vi "Teleop.vi"(8 "Enum In":enum16{"Scale", "Switch", "Intake", "Reserve"}(ring), 10 "Match Info":T1={"Autonomous Elapsed Seconds"=0.0, "TeleOp Elapsed Seconds"=0.0, "Disabled Elapsed Seconds"=0.0, "Visited Autonomous"=FALSE, "Visited TeleOp"=FALSE, "Visited Disabled"=FALSE, "Autonomous Settings"={"Autonomous Style"=enum."Independent", "VI Refnum"=refnum}}, 11 "Call Context":T2) -> (0 "Enum Out":enum16{"Scale", "Switch", "Intake", "Reserve"}(ring))   [LabVIEW 2017]
doc: "This VI is called for each enabled TeleOp packet received from the DS. It is typically used to read from joysticks and other inputs and update I/O or setpoints for timed control loops. It should complete and return within 20 milliseconds or risk missing DS packets."
uses:
  <vilib>/Rock Robotics/WPI/DriverStation/WPI_DriverStationDerivedRobotMode.ctl
  <vilib>/Rock Robotics/WPI/DriverStation/WPI_DriverStationMatch Info.ctl
  9a3754dc-426d-418a-b166-45fb967c4ccf.vi
  c9379947-65ce-468e-b721-daf5d8b91ee4.vi
  b6a63361-7184-4aa3-88ad-815ff18ec719.vi
  9926fa97-c3d7-4492-8b20-f5ff4f16c79e.vi
  7ab30a6b-1479-45e7-bda8-42199c1e9ef9.vi
  <vilib>/Rock Robotics/WPI/Utilities/WPI_GetSetVariantRefNum.vi
  <vilib>/Rock Robotics/WPI/Joystick/WPI_JoystickArcadeMapping.vi
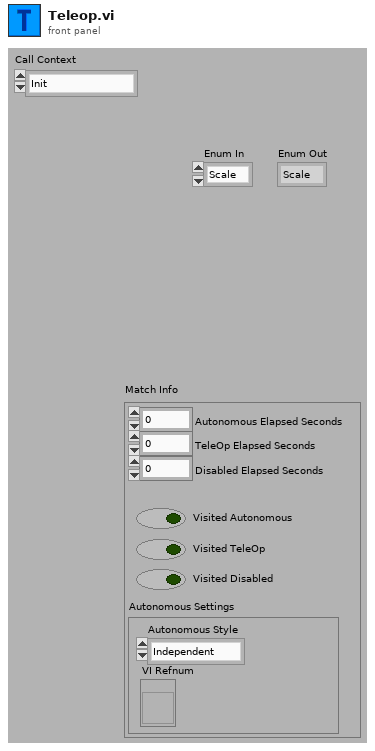
[diagram p1: front panel]
types:
  T1 = typedef "WPI_DriverStationMatch Info.ctl" = cluster{"Autonomous Elapsed Seconds":dbl, "TeleOp Elapsed Seconds":dbl, "Disabled Elapsed Seconds":dbl, "Visited Autonomous":bool, "Visited TeleOp":bool, "Visited Disabled":bool, "Autonomous Settings":cluster{"Autonomous Style":enum16{"Iterative", "Independent"}, "VI Refnum":refnum<vi>}}
  T2 = typedef "WPI_DriverStationDerivedRobotMode.ctl" = enum16{"Init", "Execute", "Stop"}
  T3 = typedef "WPI_JoystickDevRef.ctl" = cluster{"Device":T4}
  T4 = typedef "WPI_JoystickDeviceEnum.ctl" = enum16{"USB 0", "USB 1", "USB 2", "USB 3", "USB 4", "USB 5"}
  T5 = cluster{"Buttons[0]":bool, "Buttons[1]":bool, "Buttons[2]":bool, "Buttons[3]":bool, "Buttons[4]":bool, "Buttons[5]":bool, "Buttons[6]":bool, "Buttons[7]":bool, "Buttons[8]":bool}
  T6 = cluster{"POVs[0]":i16, "POVs[1]":i16, "POVs[2]":i16, "POVs[3]":i16, "POVs[4]":i16, "POVs[5]":i16, "POVs[6]":i16, "POVs[7]":i16, "POVs[8]":i16}
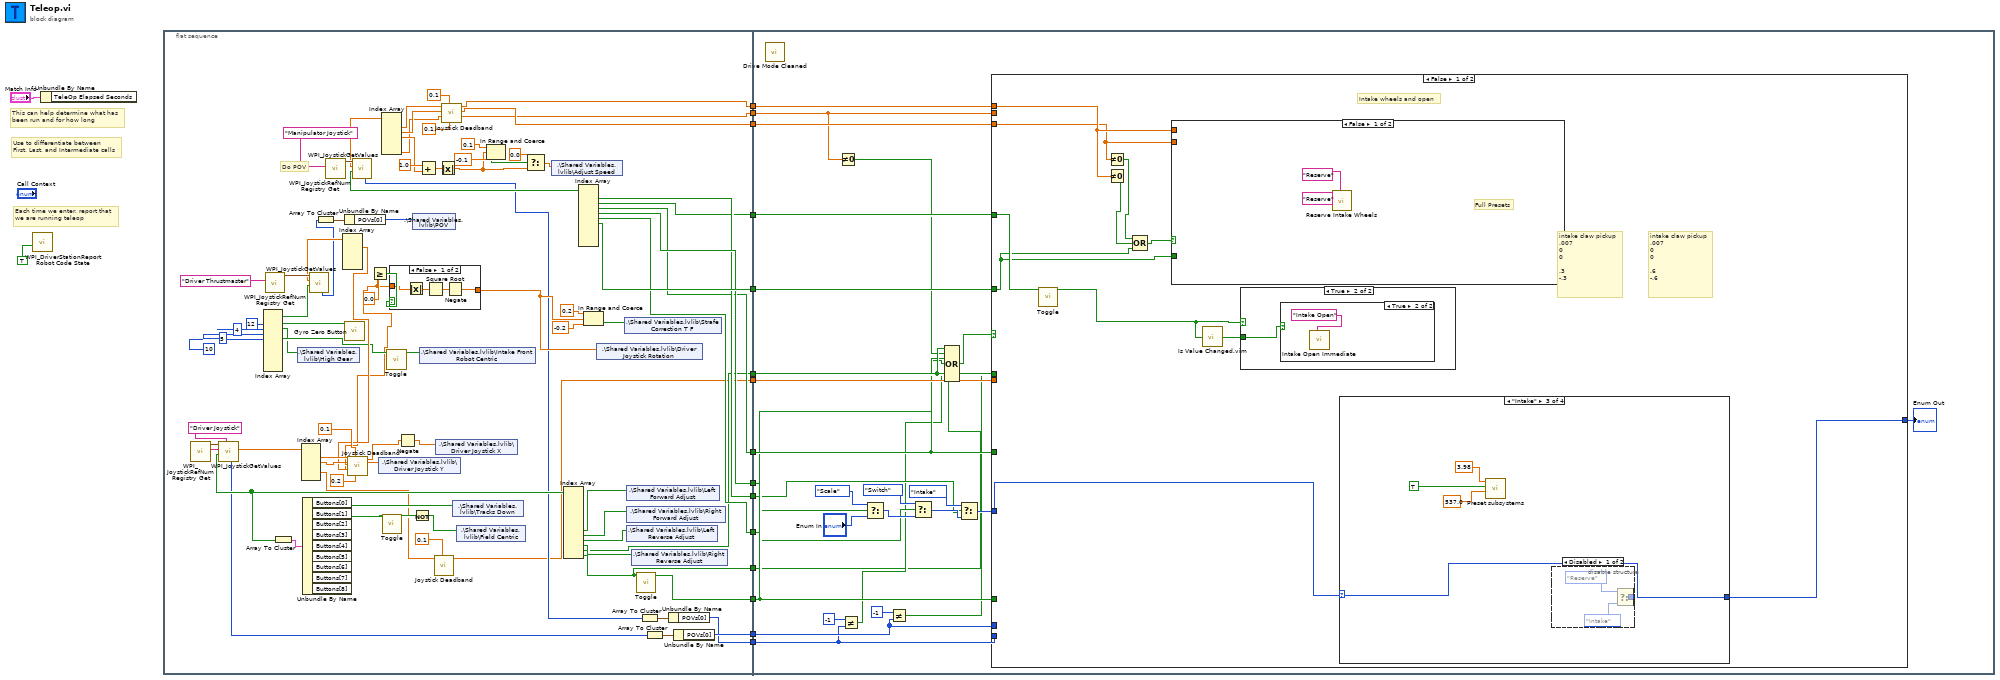
[diagram p0: block diagram]
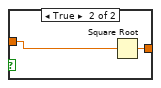
[diagram p2: hidden frame]
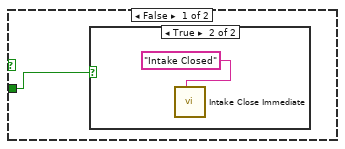
[diagram p3: hidden frame]
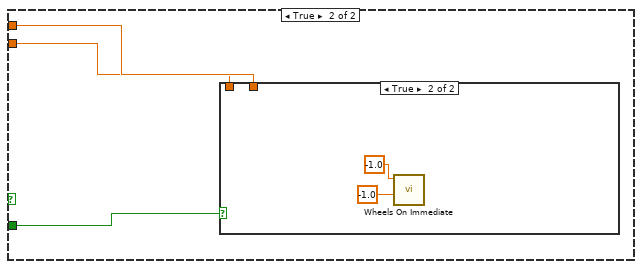
[diagram p6: hidden frame]
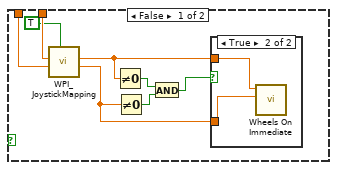
[diagram p7: hidden frame]
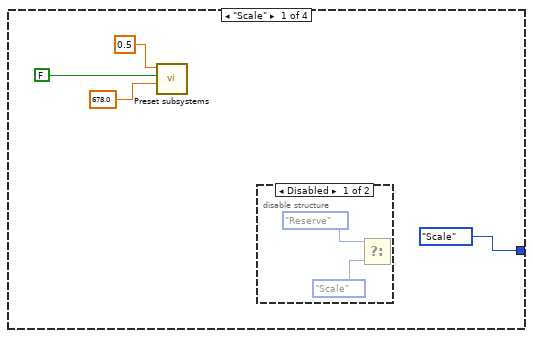
[diagram p9: hidden frame]
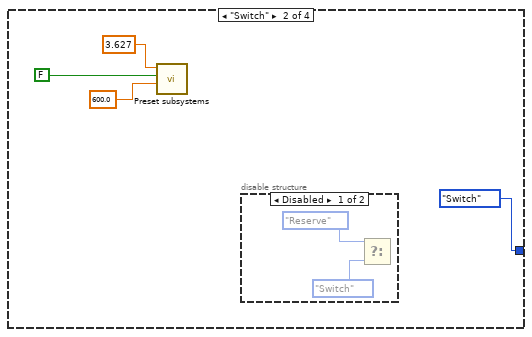
[diagram p11: hidden frame]
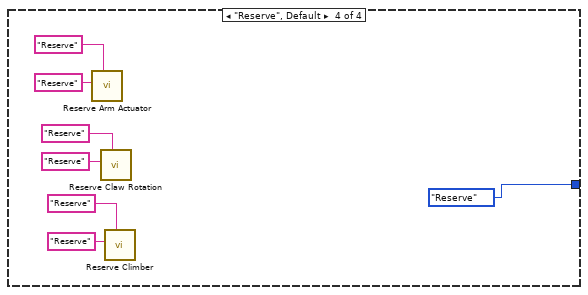
[diagram p14: hidden frame]
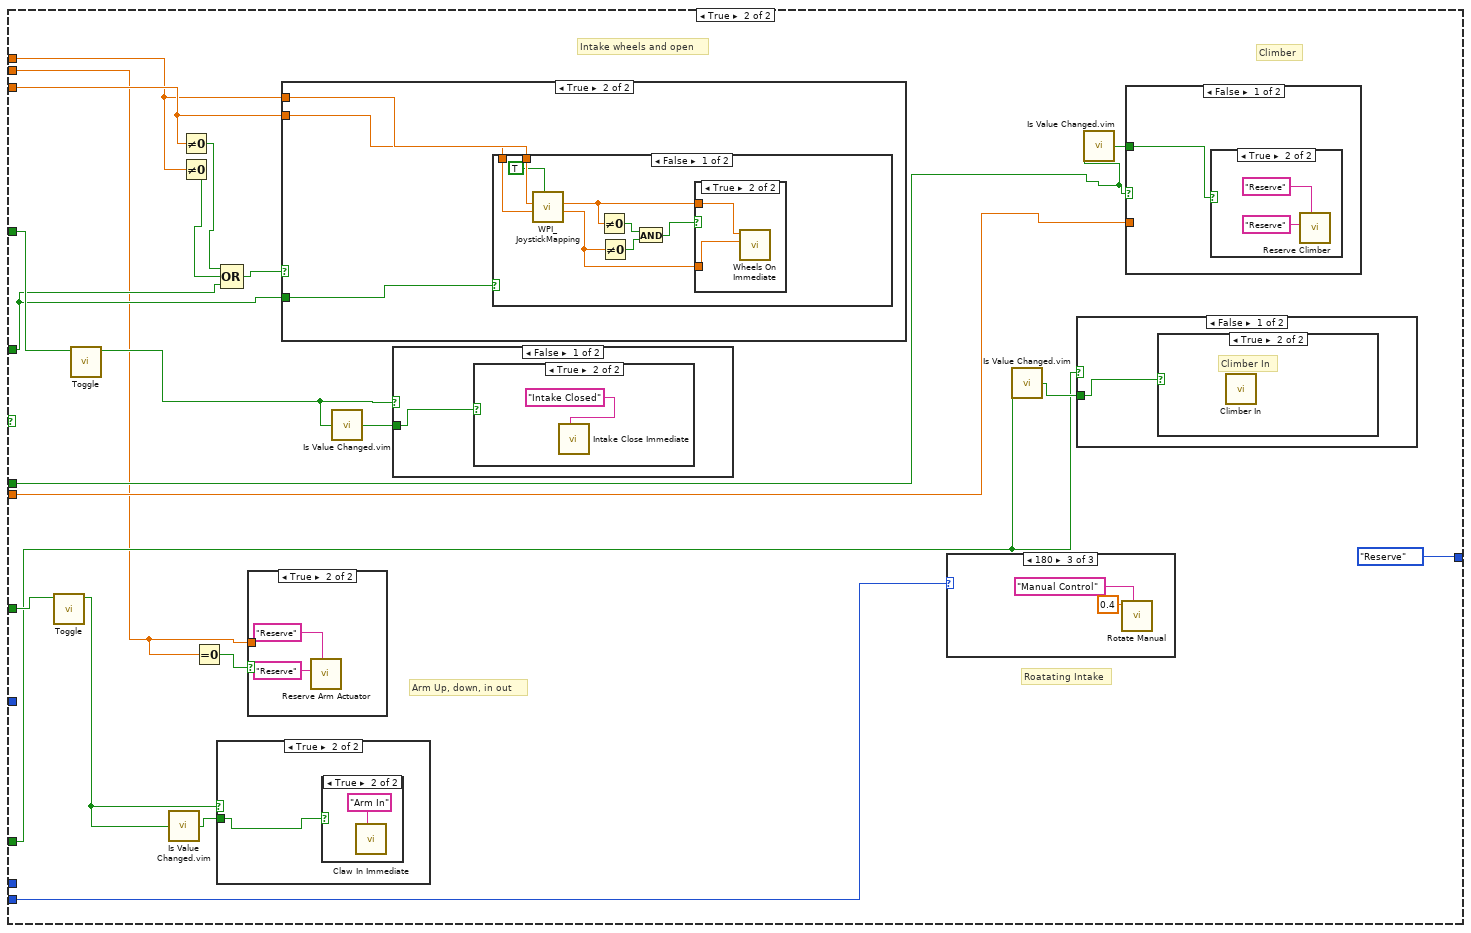
[diagram p15: hidden frame]
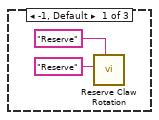
[diagram p16: hidden frame]
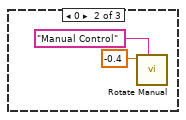
[diagram p17: hidden frame]
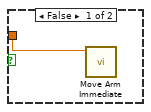
[diagram p18: hidden frame]
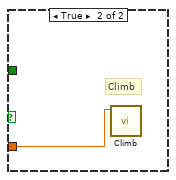
[diagram p20: hidden frame]
diagram:
  # "Each time we enter, report that\nwe are running teleop"
  # "Use to differentiate between\nFirst, Last, and Intermediate calls"
  # "This can help determine what has\nbeen run and for how long"
  n1 = call <vilib>:"WPI_DriverStationReport Robot Code State.vi"("TeleOp"=TRUE ("Autonomous")) -> ()  [unwired: 10 in, 1 out]
  n2 = Unbundle By Name("Match Info") -> ()  [unwired: 1 out]
  n3 = flat-sequence {
    tunnel: [w50] -> w15
    tunnel: [w37] -> w14
    tunnel: [w34] -> w13
    tunnel: [w33] -> w12
    tunnel: [w39] -> w11
    tunnel: [w38] -> w10
    tunnel: [w45] -> w9
    tunnel: [w41] -> w8
    tunnel: [w40] -> w7
    tunnel: [w29] -> w6
    tunnel: [w28] -> w5
    tunnel: [w23] -> w4
    tunnel: [w20] -> w3
    tunnel: [w22] -> w2
    tunnel: [w18] -> w1
    tunnel: w15 -> [w122]
    tunnel: w14 -> [w130]
    tunnel: w13 -> [w132]
    tunnel: w12 -> [w131]
    tunnel: w11 -> [w129]
    tunnel: w10 -> [w124]
    tunnel: w9 -> [w128]
    tunnel: w8 -> [w113]
    tunnel: w7 -> [w112]
    tunnel: w6 -> [w109]
    tunnel: w5 -> [w111]
    tunnel: w4 -> [w123]
    tunnel: w3 -> [w125]
    tunnel: w2 -> [w126]
    tunnel: w1 -> [w106]
    frame #0 {
      # "Do POV"
      n4 = call <vilib>:"WPI_JoystickRefNum Registry Get.vi"("refnum name"="Driver Joystick") -> ("JoystickDevRef"=w99:T3)  [unwired: 1 in, 9 out]
      n5 = call <vilib>:"WPI_JoystickGetValues.vi"("JoystickDevRef"=w99) -> ("Buttons"=w73:bool[], "Axes"=w97:dbl[], "POVs"=w51:i16[])  [unwired: 6 in, 2 out]
      n6 = call <vilib>:"WPI_JoystickRefNum Registry Get.vi"("refnum name"="Driver Thrustmaster") -> ("JoystickDevRef"=w83:T3)  [unwired: 9 in, 1 out]
      n7 = Array To Cluster(array=w73) -> (cluster=w96:T5)
      n8 = Index Array(array=w97) -> (element #1=w88:dbl, element #2=w87:dbl, element #4=w21:dbl)  [unwired: 5 in, 2 out]
      n9 = Unbundle By Name(w96) -> ("Buttons[0]"=w85:bool, "Buttons[1]"=w89:bool)  [unwired: 7 out]
      n10 = call <vilib>:"WPI_JoystickGetValues.vi"("JoystickDevRef"=w83) -> ("Buttons"=w63:bool[], "Axes"=w82:dbl[], "POVs"=w53:i16[])  [unwired: 6 in, 2 out]
      n11 = Index Array(array=w63, index #1=12 ("index"), index #2=4 ("index"), index #3=5 ("index"), index #4=10 ("index")) -> (element #1=w61:bool, element #2=w32:bool, element #4=w54:bool)  [unwired: 6 in, 7 out]
      n12 = shared-variable ".\\Shared Variables.lvlib\\High Gear"(w32) -> ()  [unwired: 1 in, 1 out]
      n13 = Array To Cluster(array=w53) -> (cluster=w58:T6)
      n14 = call <vilib>:"WPI_JoystickRefNum Registry Get.vi"("refnum name"="Manipulator Joystick") -> ("JoystickDevRef"=w94:T3)  [unwired: 1 in, 9 out]
      n15 = Index Array(array=w82) -> (element #1=w66:dbl)  [unwired: 5 in, 4 out]
      n16 = Unbundle By Name(w58) -> ("POVs[0]"=w57:i16)
      n17 = call "Gyro Zero Button.vi"("Boolean"=w61) -> ()  [unwired: 11 in]
      n18 = call "Joystick Deadband.vi"("Z Deadband"=0.2, "X Y Deadband"=0.1, "Z"=w66, "Y"=w87, "X"=w88) -> ("Z Out"=w44:dbl, "Y Out"=w92:dbl, "X Out"=w43:dbl)  [unwired: 4 in]
      n19 = call <vilib>:"WPI_JoystickGetValues.vi"("JoystickDevRef"=w94) -> ("Buttons"=w90:bool[], "Axes"=w78:dbl[], "POVs"=w30:i16[])  [unwired: 6 in, 2 out]
      n20 = Greater Or Equal?(x=w44, y=0.0) -> (x >= y?=w68:bool)
      n21 = shared-variable ".\\Shared Variables.lvlib\\Driver Joystick Y"(w92) -> ()  [unwired: 1 in, 1 out]
      n22 = Index Array(array=w78) -> (element #1=w48:dbl, element #2=w36:dbl, element #3=w69:dbl, element #6=w35:dbl)  [unwired: 6 in, 2 out]
      n23 = call "Toggle.vi"("Input"=w89) -> ("Output"=w91:bool)  [unwired: 9 in, 1 out]
      n24 = call "Toggle.vi"("Input"=w54) -> ("Output"=w55:bool)  [unwired: 9 in, 1 out]
      n25 = case shown="False" w68 {
        tunnel: [w101 w105] -> w65
        tunnel: w44 -> [w100 w104]
        frame False {
          n26 = Absolute Value(x=w100) -> (abs(x)=w103:dbl)
          n27 = Square Root(x=w103) -> (sqrt(x)=w102:dbl)
          n28 = Negate(x=w102) -> (-x=w101:dbl)
        }
        frame True {
          n29 = Square Root(x=w104) -> (sqrt(x)=w105:dbl)
        }
      }
      n30 = Negate(x=w43) -> (-x=w42:dbl)
      n31 = shared-variable ".\\Shared Variables.lvlib\\POV"(w57) -> ()  [unwired: 1 in, 1 out]
      n32 = Not(x=w91) -> (.not. x?=w86:bool)
      n33 = Add(x=1.0, y=w69) -> (x+y=w72:dbl)
      n34 = shared-variable ".\\Shared Variables.lvlib\\Intake Front Robot Centric"(w55) -> ()  [unwired: 1 in, 1 out]
      n35 = call "Joystick Deadband.vi"("X Y Deadband"=0.1, "X"=w21) -> ("X Out"=w20:dbl)  [unwired: 7 in, 2 out]
      n36 = shared-variable ".\\Shared Variables.lvlib\\Driver Joystick X"(w42) -> ()  [unwired: 1 in, 1 out]
      n37 = Absolute Value(x=w72) -> (abs(x)=w70:dbl)
      n38 = call "Joystick Deadband.vi"("Z Deadband"=0.1, "X Y Deadband"=0.1, "Z"=w35, "Y"=w36, "X"=w48) -> ("Z Out"=w33:dbl, "Y Out"=w34:dbl, "X Out"=w37:dbl)  [unwired: 4 in]
      n39 = shared-variable ".\\Shared Variables.lvlib\\Tracks Down"(w85) -> ()  [unwired: 1 in, 1 out]
      n40 = shared-variable ".\\Shared Variables.lvlib\\Field Centric"(w86) -> ()  [unwired: 1 in, 1 out]
      n41 = In Range and Coerce(upper limit=0.1, x=w70, lower limit=-0.1 ("x")) -> (In Range?=w75:bool)  [unwired: 1 out]
      n42 = Select(t=0.0, s=w75, f=w70) -> (s? t:f=w64:dbl)
      n43 = shared-variable ".\\Shared Variables.lvlib\\Adjust Speed"(w64) -> ()  [unwired: 1 in, 1 out]
      n44 = Index Array(array=w73) -> (element #7=w27:bool, element #8=w26:bool, element #9=w25:bool, element #10=w24:bool, element #11=w22:bool, element #12=w18:bool)  [unwired: 12 in, 6 out]
      n45 = Index Array(array=w90) -> (element #1=w40:bool, element #2=w39:bool, element #3=w38:bool, element #4=w41:bool, element #5=w28:bool, element #6=w45:bool)  [unwired: 10 in, 4 out]
      n46 = In Range and Coerce(upper limit=0.2, x=w65, lower limit=-0.2) -> (In Range?=w81:bool)  [unwired: 1 out]
      n47 = shared-variable ".\\Shared Variables.lvlib\\Driver Joystick Rotation"(w65) -> ()  [unwired: 1 in, 1 out]
      n48 = shared-variable ".\\Shared Variables.lvlib\\Strafe Correction T F"(w81) -> ()  [unwired: 1 in, 1 out]
      n49 = shared-variable ".\\Shared Variables.lvlib\\Left Forward Adjust"(w27) -> ()  [unwired: 1 in, 1 out]
      n50 = shared-variable ".\\Shared Variables.lvlib\\Left Reverse Adjust"(w25) -> ()  [unwired: 1 in, 1 out]
      n51 = shared-variable ".\\Shared Variables.lvlib\\Right Forward Adjust"(w26) -> ()  [unwired: 1 in, 1 out]
      n52 = shared-variable ".\\Shared Variables.lvlib\\Right Reverse Adjust"(w24) -> ()  [unwired: 1 in, 1 out]
      n53 = call "Toggle.vi"("Input"=w18) -> ("Output"=w23:bool)  [unwired: 9 in, 1 out]
      n54 = Array To Cluster(array=w30) -> (cluster=w31:T6)
      n55 = Array To Cluster(array=w51) -> (cluster=w52:T6)
      n56 = Unbundle By Name(w31) -> ("POVs[0]"=w29:i16)
      n57 = Unbundle By Name(w52) -> ("POVs[0]"=w50:i16)
    }
    frame #1 {
      n58 = call "Drive Mode Cleaned.vi"() -> ()  [unwired: 12 in]
      n59 = Not Equal To 0?(x=w131) -> (x != 0?=w107:bool)
      n60 = Not Equal?(x=i16 -1, y=w109) -> (x != y?=w108:bool)
      n61 = Select(t=enum16{"Scale", "Switch", "Intake", "Reserve"}."Scale", s=w113, f="Enum In") -> (s? t:f=w116:enum16{"Scale", "Switch", "Intake", "Reserve"})
      n62 = Not Equal?(x=i16 -1, y=w122) -> (x != y?=w120:bool)
      n63 = Select(t=enum16{"Scale", "Switch", "Intake", "Reserve"}."Switch", s=w111, f=w116) -> (s? t:f=w114:enum16{"Scale", "Switch", "Intake", "Reserve"})
      n64 = Compound Arithmetic op=OR(w126, w107, w124, w123, w120, w108, w106) -> (w127:bool)
      n65 = Select(t=enum16{"Scale", "Switch", "Intake", "Reserve"}."Intake", s=w112, f=w114) -> (s? t:f=w133:enum16{"Scale", "Switch", "Intake", "Reserve"})
      n66 = case shown="False" w127 {
        tunnel: w131 -> [_ w193]
        tunnel: w129 -> [w138 w213]
        tunnel: w122 -> [_ _]
        tunnel: w132 -> [w136 w212]
        tunnel: w130 -> [w137 w211]
        tunnel: w128 -> [w135 w194]
        tunnel: w124 -> [_ w210]
        tunnel: w109 -> [_ w202]
        tunnel: w123 -> [_ w200]
        tunnel: w125 -> [_ w198]
        tunnel: w126 -> [_ w197]
        tunnel: [w145 enum16{"Scale", "Switch", "Intake", "Reserve"}."Reserve"] -> w134
        tunnel: w133 -> [w144 _]
        frame False {
          # "Intake wheels and open"
          # "intake claw pickup\n.007\n0\n0\n\n.6\n-.6"
          # "intake claw pickup\n.007\n0\n0\n\n.3\n-.3"
          # "Full Presets"
          n67 = call "Toggle.vi"("Input"=w138) -> ("Output"=w139:bool)  [unwired: 9 in, 1 out]
          n68 = Not Equal To 0?(x=w136) -> (x != 0?=w140:bool)
          n69 = Not Equal To 0?(x=w137) -> (x != 0?=w141:bool)
          n70 = Compound Arithmetic op=OR(w140, w141, w135) -> (w142:bool)
          n71 = case shown="False" w142 {
            tunnel: w137 -> [_ w154]
            tunnel: w136 -> [_ w153]
            tunnel: w135 -> [_ w152]
            frame False {
              n72 = call "Reserve Intake Wheels.vi"("Description"="Reserve", "Command Name"="Reserve") -> ()  [unwired: 9 in, 1 out]
            }
            frame True {
              n73 = case shown="True" w152 {
                tunnel: w154 -> [w159 _]
                tunnel: w153 -> [w158 _]
                frame False {
                  n74 = call-poly <vilib>:"WPI_JoystickMapping.vi"("Square Inputs"=TRUE, "Y axis value"=w158, "X axis value"=w159) -> ("Right Motor Value"=w155:dbl, "Left Motor Value"=w156:dbl)  [unwired: 7 in]
                  n75 = Not Equal To 0?(x=w156) -> (x != 0?=w162:bool)
                  n76 = Not Equal To 0?(x=w155) -> (x != 0?=w161:bool)
                  n77 = And(x=w162, y=w161) -> (x .and. y?=w160:bool)
                  n78 = case shown="True" w160 {
                    tunnel: w156 -> [_ w164]
                    tunnel: w155 -> [_ w163]
                    frame False {
                    }
                    frame True {
                      n79 = call "Wheels On Immediate.vi"("Right Wheel"=w163, "Left Wheel"=w164) -> ()  [unwired: 9 in, 1 out]
                    }
                  }
                }
                frame True {
                  n80 = call "Wheels On Immediate.vi"("Right Wheel"=-1.0, "Left Wheel"=-1.0) -> ()  [unwired: 9 in, 1 out]
                }
              }
            }
          }
          n81 = call "Is Value Changed.vim"("value"=w139) -> ("changed or first call?"=w143:bool)
          n82 = case shown="True" w139 {
            tunnel: w143 -> [w146 w148]
            frame False {
              n83 = case shown="True" w146 {
                frame False {
                }
                frame True {
                  n84 = call "Intake Close Immediate.vi"("Description"="Intake Closed") -> ()  [unwired: 10 in, 1 out]
                }
              }
            }
            frame True {
              n85 = case shown="True" w148 {
                frame False {
                }
                frame True {
                  n86 = call "Intake Open Immediate.vi"("Description"="Intake Open") -> ()  [unwired: 10 in, 1 out]
                }
              }
            }
          }
          n87 = case shown="\"Intake\"" w144 {
            selector: w144 -> [_ _ w179 _]
            tunnel: [enum16{"Scale", "Switch", "Intake", "Reserve"}."Scale" enum16{"Scale", "Switch", "Intake", "Reserve"}."Switch" w179 enum16{"Scale", "Switch", "Intake", "Reserve"}."Reserve"] -> w145
            frame "Scale" {
              n88 = call "Preset subsystems.vi"("Claw Angle"=678.0, "Arm Extend?"=FALSE, "Arm Angle"=0.5) -> ()  [unwired: 9 in]
              n89 = disable-structure shown="Disabled" {
                frame Disabled {
                  n90 = Select(t=enum16{"Scale", "Switch", "Intake", "Reserve"}."Reserve", f=enum16{"Scale", "Switch", "Intake", "Reserve"}."Scale") -> ()  [unwired: 1 in, 1 out]
                }
                frame Enabled {
                }
              }
            }
            frame "Switch" {
              n91 = call "Preset subsystems.vi"("Claw Angle"=600.0, "Arm Extend?"=FALSE, "Arm Angle"=3.627) -> ()  [unwired: 9 in]
              n92 = disable-structure shown="Disabled" {
                frame Disabled {
                  n93 = Select(t=enum16{"Scale", "Switch", "Intake", "Reserve"}."Reserve", f=enum16{"Scale", "Switch", "Intake", "Reserve"}."Switch") -> ()  [unwired: 1 in, 1 out]
                }
                frame Enabled {
                }
              }
            }
            frame "Intake" {
              n94 = call "Preset subsystems.vi"("Claw Angle"=537.0, "Arm Extend?"=TRUE, "Arm Angle"=3.98) -> ()  [unwired: 9 in]
              n95 = disable-structure shown="Disabled" {
                disable-tunnel: [w183 _] -> _
                frame Disabled {
                  n96 = Select(t=enum16{"Scale", "Switch", "Intake", "Reserve"}."Reserve", f=enum16{"Scale", "Switch", "Intake", "Reserve"}."Intake") -> (s? t:f=w183:enum16{"Scale", "Switch", "Intake", "Reserve"})  [unwired: 1 in]
                }
                frame Enabled {
                }
              }
            }
            frame "Reserve", Default {
              n97 = call "Reserve Arm Actuator.vi"("Description"="Reserve", "Command Name"="Reserve") -> ()  [unwired: 9 in, 1 out]
              n98 = call "Reserve Claw Rotation.vi"("Description"="Reserve", "Command Name"="Reserve") -> ()  [unwired: 9 in, 1 out]
              n99 = call "Reserve Climber.vi"("Description"="Reserve", "Command Name"="Reserve") -> ()  [unwired: 9 in, 1 out]
            }
          }
        }
        frame True {
          # "Arm Up, down, in out"
          # "Intake wheels and open"
          # "Roatating Intake"
          # "Climber"
          n100 = call "Toggle.vi"("Input"=w210) -> ("Output"=w203:bool)  [unwired: 9 in, 1 out]
          n101 = call "Toggle.vi"("Input"=w213) -> ("Output"=w209:bool)  [unwired: 9 in, 1 out]
          n102 = call "Is Value Changed.vim"("value"=w203) -> ("changed or first call?"=w204:bool)
          n103 = Not Equal To 0?(x=w212) -> (x != 0?=w208:bool)
          n104 = Not Equal To 0?(x=w211) -> (x != 0?=w207:bool)
          n105 = Equal To 0?(x=w193) -> (x = 0?=w195:bool)
          n106 = case shown="True" w203 {
            tunnel: w204 -> [w229 w231]
            frame False {
              n107 = case shown="True" w229 {
                frame False {
                }
                frame True {
                  n108 = call "Claw Out Immediate.vi"("Description"="Arm Out") -> ()  [unwired: 10 in, 1 out]
                }
              }
            }
            frame True {
              n109 = case shown="True" w231 {
                frame False {
                }
                frame True {
                  n110 = call "Claw In Immediate.vi"("Description"="Arm In") -> ()  [unwired: 10 in, 1 out]
                }
              }
            }
          }
          n111 = Compound Arithmetic op=OR(w208, w207, w194) -> (w206:bool)
          n112 = case shown="True" w195 {
            tunnel: w193 -> [w220 _]
            frame False {
              n113 = call "Move Arm Immediate.vi"("Arm Speed"=w220) -> ()  [unwired: 10 in, 1 out]
            }
            frame True {
              n114 = call "Reserve Arm Actuator.vi"("Description"="Reserve", "Command Name"="Reserve") -> ()  [unwired: 9 in, 1 out]
            }
          }
          n115 = case shown="True" w206 {
            tunnel: w211 -> [_ w241]
            tunnel: w212 -> [_ w240]
            tunnel: w194 -> [_ w239]
            frame False {
              n116 = call "Reserve Intake Wheels.vi"("Description"="Reserve", "Command Name"="Reserve") -> ()  [unwired: 9 in, 1 out]
            }
            frame True {
              n117 = case shown="False" w239 {
                tunnel: w241 -> [w246 _]
                tunnel: w240 -> [w245 _]
                frame False {
                  n118 = call-poly <vilib>:"WPI_JoystickMapping.vi"("Square Inputs"=TRUE, "Y axis value"=w245, "X axis value"=w246) -> ("Right Motor Value"=w242:dbl, "Left Motor Value"=w243:dbl)  [unwired: 7 in]
                  n119 = Not Equal To 0?(x=w243) -> (x != 0?=w249:bool)
                  n120 = Not Equal To 0?(x=w242) -> (x != 0?=w248:bool)
                  n121 = And(x=w249, y=w248) -> (x .and. y?=w247:bool)
                  n122 = case shown="True" w247 {
                    tunnel: w243 -> [_ w251]
                    tunnel: w242 -> [_ w250]
                    frame False {
                    }
                    frame True {
                      n123 = call "Wheels On Immediate.vi"("Right Wheel"=w250, "Left Wheel"=w251) -> ()  [unwired: 9 in, 1 out]
                    }
                  }
                }
                frame True {
                  n124 = call "Wheels On Immediate.vi"("Right Wheel"=-1.0, "Left Wheel"=-1.0) -> ()  [unwired: 9 in, 1 out]
                }
              }
            }
          }
          n125 = call "Is Value Changed.vim"("value"=w209) -> ("changed or first call?"=w205:bool)
          n126 = case shown="False" w209 {
            tunnel: w205 -> [w233 w235]
            frame False {
              n127 = case shown="True" w233 {
                frame False {
                }
                frame True {
                  n128 = call "Intake Close Immediate.vi"("Description"="Intake Closed") -> ()  [unwired: 10 in, 1 out]
                }
              }
            }
            frame True {
              n129 = case shown="True" w235 {
                frame False {
                }
                frame True {
                  n130 = call "Intake Open Immediate.vi"("Description"="Intake Open") -> ()  [unwired: 10 in, 1 out]
                }
              }
            }
          }
          n131 = case shown="180" w202 {
            frame -1, Default {
              n132 = call "Reserve Claw Rotation.vi"("Description"="Reserve", "Command Name"="Reserve") -> ()  [unwired: 9 in, 1 out]
            }
            frame 0 {
              n133 = call "Rotate Manual.vi"("Description"="Manual Control", "Setpoint"=-0.4) -> ()  [unwired: 9 in, 1 out]
            }
            frame 180 {
              n134 = call "Rotate Manual.vi"("Description"="Manual Control", "Setpoint"=0.4) -> ()  [unwired: 9 in, 1 out]
            }
          }
          n135 = call "Is Value Changed.vim"("value"=w200) -> ("changed or first call?"=w201:bool)
          n136 = case shown="False" w200 {
            tunnel: w201 -> [w227 w228]
            frame False {
              n137 = case shown="True" w227 {
                frame False {
                }
                frame True {
                  # "Climber In"
                  n138 = call "Climber In.vi"() -> ()  [unwired: 11 in, 1 out]
                }
              }
            }
            frame True {
              n139 = case shown="True" w228 {
                frame False {
                }
                frame True {
                  # "Climber Out"
                  n140 = call "Climber Out.vi"() -> ()  [unwired: 11 in, 1 out]
                }
              }
            }
          }
          n141 = call "Is Value Changed.vim"("value"=w197) -> ("changed or first call?"=w199:bool)
          n142 = case shown="False" w197 {
            tunnel: w199 -> [w223 _]
            tunnel: w198 -> [_ w226]
            frame False {
              n143 = case shown="True" w223 {
                frame False {
                }
                frame True {
                  n144 = call "Reserve Climber.vi"("Description"="Reserve", "Command Name"="Reserve") -> ()  [unwired: 9 in, 1 out]
                }
              }
            }
            frame True {
              # "Climb"
              n145 = call "Climb.vi"("Driver Stick Y"=w226) -> ()  [unwired: 10 in, 1 out]
            }
          }
        }
      }
      "Enum Out" <- w134
    }
  }
